vi "Power OFF-Ganging.vi"(8 "error in":errorcluster, 9 "Ganged Config":T1, 10 "Slave resource names":string[](array[string]), 11 "Master resouce name":string) -> (3 "Status":string)   [LabVIEW 2021]
doc: "This VI will reset the source and load devices, which results in powering off the DUT for stacked/ganged-channel configuration."
uses:
  channel ganging/shared subVIs/ctl/NIDCPower_channel_ganging - ctl - ganged config.ctl
panel:
  out "error out":errorcluster
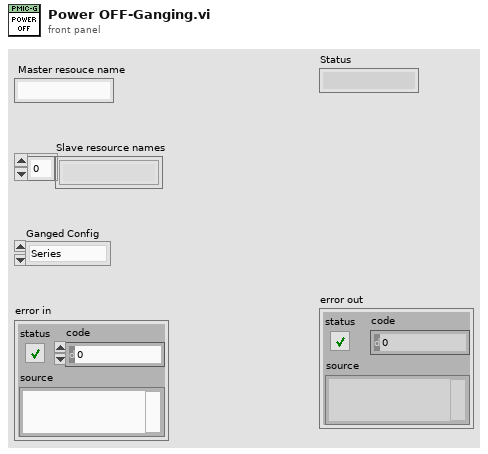
[diagram p1: front panel]
types:
  T1 = typedef "NIDCPower_channel_ganging - ctl - ganged config.ctl" = enum32{"Series", "Parallel", "Manual"}
  T2 = typedef "NIDCPower_channel_ganging - ctl - channel def.ctl" = cluster{"resource name":refnum<k15>, "channels":string, "Channel Mode":T3}
  T3 = typedef "NIDCPower_channel_ganging - ctl - channel mode.ctl" = enum32{"Master", "Slave", "Slave - Inverted"}
  T4 = typedef "NIDCPower_channel_ganging - ctl - ganged session.ctl" = cluster{"Ganged Config":T1, "Session List":refnum<k15>[], "Session Mode":T3[], "Channel":string[]}
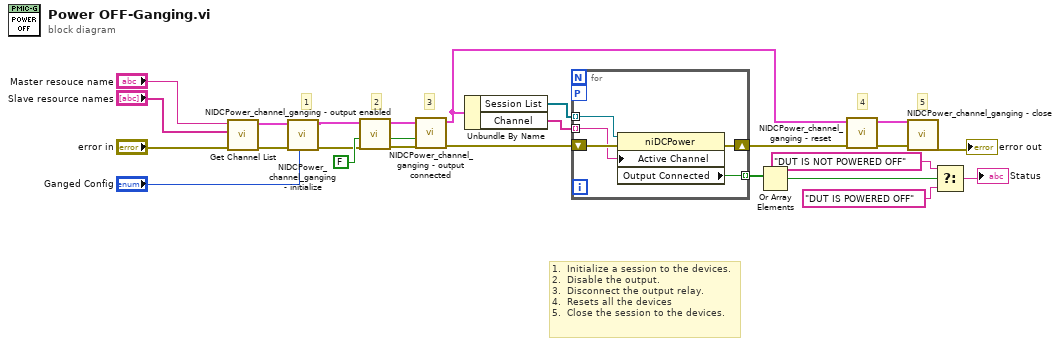
[diagram p0: block diagram]
diagram:
  w16 = FALSE ("output enabled")
  # "5"
  # "4"
  # "3"
  # "2"
  # "1"
  # "1.  Initialize a session to the devices.\n2.  Disable the output.\n3.  Disconnect the output relay.\n4.  Resets all the devices\n5.  Close the session to the devices."
  n1 = call "Get Channel List.vi"("error in (no error)"="error in", "Slave resource names"="Slave resource names", "Master resouce name"="Master resouce name") -> ("error out"=w23:errorcluster, "Channel List"=w24:T2[])  [unwired: 7 in]
  n2 = call "NIDCPower_channel_ganging - initialize.vi"("Ganged Config"="Ganged Config", "error in (no error)"=w23, "Channel List"=w24) -> ("error out"=w13:errorcluster, "Ganged Session Out"=w12:T4)  [unwired: 7 in]
  n3 = call "NIDCPower_channel_ganging - output enabled.vi"("error in (no error)"=w13, "output enabled"=w16, "Ganged Session In"=w12) -> ("error out"=w18:errorcluster, "Ganged Session Out"=w17:T4)  [unwired: 7 in]
  n4 = call "NIDCPower_channel_ganging - output connected.vi"("error in (no error)"=w18, "output enabled"=w16, "Ganged Session In"=w17) -> ("error out"=w8:errorcluster, "Ganged Session Out"=w6:T4)  [unwired: 7 in]
  n5 = Unbundle By Name(w6) -> ("Session List"=w10:refnum<k15>[], "Channel"=w9:string[])
  n6 = for {
    shift-right: [w27] -> w7
    shift-left: w8 -> [w28]
    tunnel: w10 -> [w29] mode=indexing
    workers-P: _ -> [_]
    tunnel: w9 -> [w26] mode=indexing
    tunnel: [w25] -> w2 mode=indexing
    n7 = property class="niDCPower"(reference=w29, error in=w28, "Active Channel"=w26) -> (error out=w27:errorcluster, "Output Connected"=w25:bool)  [unwired: 1 out]
  }
  n8 = Or Array Elements(Boolean array=w2) -> (logical OR=w1:bool)
  n9 = call "NIDCPower_channel_ganging - reset.vi"("error in (no error)"=w7, "Ganged Session In"=w6) -> ("error out"=w14:errorcluster, "Ganged Session Out"=w15:T4)  [unwired: 8 in]
  n10 = call "NIDCPower_channel_ganging - close.vi"("error in (no error)"=w14, "Ganged Session In"=w15) -> ("error out"=→"error out":errorcluster)  [unwired: 9 in]
  n11 = Select(t="DUT IS NOT POWERED OFF" ("Status"), s=w1, f="DUT IS POWERED OFF" ("Status")) -> (s? t:f=→"Status":string)
